vi "Generate Victim and Interferer Waveforms.vi"(6 "hardware commands sync queue":T2, 7 "measurement configuration":T1={"Victim channel"=0, "Full scale range"=10.0, "Interferer channels"=[2], "Victim channel resource name"="", "Victim frequency"=1000.0, "Victim amplitude"=-1.0, "Interferer channel resource name"="", "Interferer channel channel"=0, "Interferer start frequency"=100000.0, "Interferer stop frequency"=160000.0, "Interferer number of steps"=10, "Interferer sweep type"=0, "Interferer amplitude"=-1.0, "Digital capture resource name"="", "Digital capture sample rate"=800000.0, "Digital capture samples"=800000} {"Interferer sweep type" items=["Linear", "Logarithmic"]}, 8 "error in":errorcluster, 10 "FGen session in":refnum<k15>, 11 "DSG task in":refnum<k21>) -> (0 "error out":errorcluster)   [LabVIEW 2021, in "adc_chToChIsolationMeasurement.lvlib"]
uses:
  adc_chToChIsolationMeasurement.lvlib
  shared/controls/HW Sync Commands Queue Ref.ctl
  shared/controls/HW Sync Commands.ctl
  Measurement Configuration.ctl
  <vilib>/addons/_NISVFA/_Generation/Signal Generation/SV Signal/sv_System Timing Model.ctl
  <vilib>/DAQmx/write.llb/DAQmx Write (Analog Wfm 1Chan NSamp).vi
  <vilib>/addons/_NISVFA/_Generation/Signal Generation/SV Sinusoid/SV Sinusoid.lvclass
  C:/Program Files/National Instruments/LabVIEW 2021/vi.lib/addons/_NISVFA/_Generation/Signal Generation/SV Signal/SV Signal.lvclass
  <vilib>/addons/_NISVFA/_Generation/Signal Generation/SV Sinusoid/Configure Sine.vi
  <vilib>/addons/_NISVFA/_Generation/Signal Generation/SV Signal/Write Sample Rate.vi
  <vilib>/addons/_NISVFA/_Generation/Signal Generation/SV Signal/Write System Timing Model.vi
  <vilib>/addons/_NISVFA/_Generation/Signal Generation/SV Signal/Write Ramp Parameters.vi
  <vilib>/DAQmx/miscellaneous.llb/DAQmx Fill In Error Info.vi
  <resource>/objmgr/daqmx.rc
  <vilib>/addons/_NISVFA/_Generation/Signal Generation/SV Signal/SV Signal.lvclass
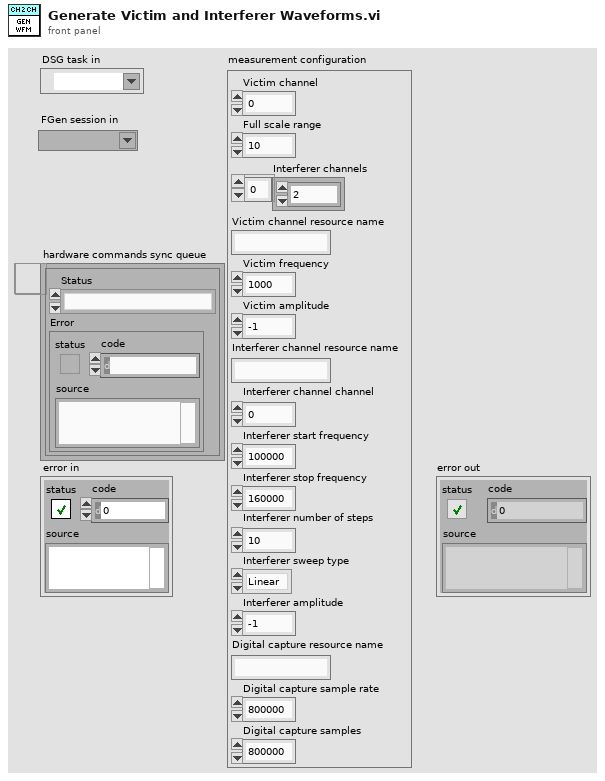
[diagram p1: front panel]
types:
  T1 = typedef "adc_chToChIsolationMeasurement.lvlib/Measurement Configuration.ctl" = cluster{"Victim channel":i32, "Full scale range":dbl, "Interferer channels":i32[], "Victim channel resource name":string, "Victim frequency":dbl, "Victim amplitude":dbl, "Interferer channel resource name":string, "Interferer channel channel":i32, "Interferer start frequency":dbl, "Interferer stop frequency":dbl, "Interferer number of steps":i32, "Interferer sweep type":u16, "Interferer amplitude":dbl, "Digital capture resource name":string, "Digital capture sample rate":dbl, "Digital capture samples":u32}
  T2 = typedef "HW Sync Commands Queue Ref.ctl" = refnum<queue>
  T3 = cluster{"profile":enum16{"Linear", "Half cosine"}, "durations [s]":cluster{"ramp-up":dbl, "transition":dbl, "ramp-down":dbl}}
  T4 = typedef "HW Sync Commands.ctl" = enum16{"NoAction", "GenerationStarted", "AcquisitionCompleted", "GenerationErrored"}
  T5 = typedef "SV Signal.lvclass/sv_System Timing Model.ctl" = i64
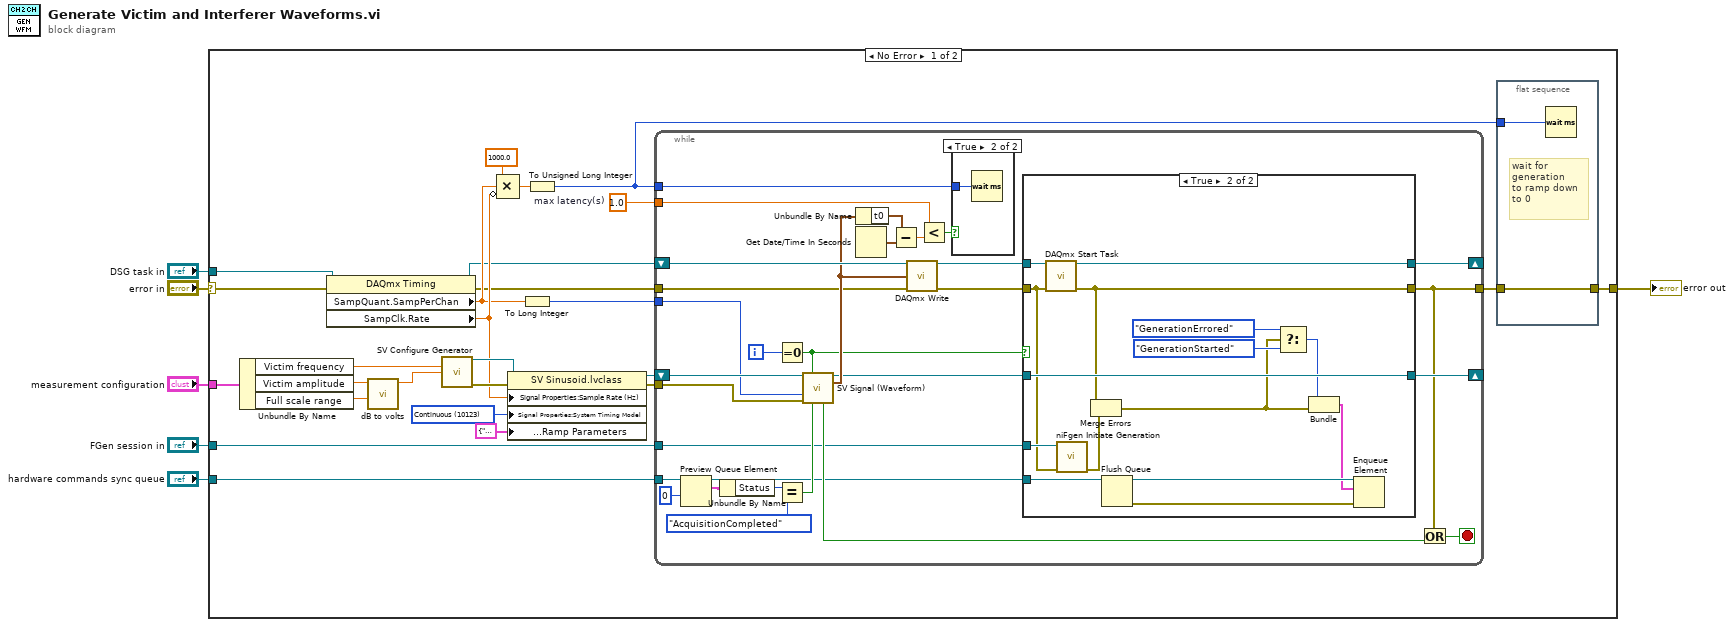
[diagram p0: block diagram]
diagram:
  n1 = case shown="No Error" "error in" {
    selector: "error in" -> [w32 w84]
    tunnel: [w31 w84] -> w5
    tunnel: "DSG task in" -> [w27 _]
    tunnel: "hardware commands sync queue" -> [w30 _]
    tunnel: "measurement configuration" -> [w29 _]
    tunnel: "FGen session in" -> [w10 _]
    frame No Error {
      w17 = 1.0  # max latency(s)
      w24 = T5 10123 items=["Finite"=10178, "-"=-1, "Continuous"=10123, "-"=-2, "Settled"=110123, "Averaged"=210123, "Discrete Sweep"=310123, "Continuous Sweep"=410123] ("System Timing Model")
      n2 = Unbundle By Name(w29) -> ("Victim frequency"=w28:dbl, "Victim amplitude"=w9:dbl, "Full scale range"=w8:dbl)
      n3 = property class="DAQmx Timing"(reference=w27, error in=w32) -> (reference out=w18:refnum<k21>, error out=w11:errorcluster, "SampQuant.SampPerChan"=w20:dbl, "SampClk.Rate"=w23:dbl)
      n4 = call "dB to volts.vi"("Full scale range"=w8, "Voltage(dB)"=w9) -> ("Voltage(volts)"=w7:dbl)  [unwired: 9 in]
      n5 = call-poly <vilib>:"SV Configure Generator.vi"("frequency (Hz)"=w28, "amplitude"=w7) -> ("signal configuration"=w25:refnum<class "SV Sinusoid.lvclass">, "error out"=w26:errorcluster)  [unwired: 12 in]
      n6 = Compound Arithmetic op=MULTIPLY(1000.0 ("value"), w20, invert w23) -> (w16:dbl)
      n7 = property class="SV Sinusoid.lvclass"(reference=w25, error in=w26, "Signal Properties:Sample Rate (Hz)"=w23, "Signal Properties:System Timing Model"=w24, "Signal Properties:Ramps:Ramp Parameters"=T3 {"profile"=enum."Linear", "durations [s]"={"ramp-up"=0.0, "transition"=0.0, "ramp-down"=0.01}} ("Ramp Parameters:All Elements")) -> (reference out=w22:refnum<class "SV Sinusoid.lvclass">, error out=w21:errorcluster)
      n8 = To Long Integer(number=w20) -> (32bit integer=w19:i32)
      n9 = To Unsigned Long Integer(number=w16) -> (unsigned 32bit integer=w13:u32)
      n10 = while {
        shift-right: [w40] -> _
        shift-left: w22 -> [w64]
        tunnel: w21 -> [w61]
        tunnel: w19 -> [w62]
        shift-right: [w43] -> _
        shift-left: w18 -> [w60]
        tunnel: [w37] -> w14
        tunnel: w17 -> [w53]
        tunnel: w13 -> [w51]
        tunnel: w30 -> [w50]
        tunnel: w11 -> [w36]
        tunnel: w10 -> [w35]
        i -> [w63]
        stop <- w58 stop-if-true
        n11 = Preview Queue Element(queue=w50, timeout in ms (-1)=0) -> (queue out=w46:T2, element=w39:cluster{"Status":T4, "Error":errorcluster})  [unwired: 1 in, 2 out]
        n12 = Unbundle By Name(w39) -> ("Status"=w38:T4)
        n13 = Equal To 0?(x=w63) -> (x = 0?=w45:bool)
        n14 = Equal?(x=w38, y=HW_Sync_Commands."AcquisitionCompleted") -> (x = y?=w47:bool)
        n15 = call-dynamic "SV Signal (Waveform).vi"("signal configuration"=w64, "reset"=w45, "samples"=w62, "error in (no error)"=w61, "stop"=w47) -> ("signal configuration"=w41:refnum<class "SV Sinusoid.lvclass">, "output waveform"=w57:waveform(dbl), "done"=w59:bool)  [unwired: 5 in, 3 out]
        n16 = Unbundle By Name(w57) -> ("t0"=w56:timestamp)
        n17 = Get Date/Time In Seconds() -> (seconds since 1Jan1904=w55:timestamp)
        n18 = Subtract(x=w56, y=w55) -> (x-y=w54:dbl)
        n19 = call-poly <vilib>:"DAQmx Write.vi"("task/channels in"=w60, "data"=w57, "error in"=w36) -> ("task out"=w44:refnum<k21>, "error out"=w42:errorcluster)  [unwired: 10 in, 1 out]
        n20 = Less?(x=w53, y=w54) -> (x < y?=w52:bool)
        n21 = case shown="True" w52 {
          tunnel: w51 -> [_ w83]
          frame False {
          }
          frame True {
            n22 = Wait (ms)(milliseconds to wait=w83) -> ()  [unwired: 1 out]
          }
        }
        n23 = case shown="True" w45 {
          tunnel: w46 -> [_ w82]
          tunnel: w44 -> [w67 w80]
          tunnel: [w67 w79] -> w43
          tunnel: w42 -> [w66 w71]
          tunnel: [w66 w69] -> w37
          tunnel: w41 -> [w65 w75]
          tunnel: [w65 w75] -> w40
          tunnel: w35 -> [_ w72]
          frame False {
          }
          frame True {
            n24 = call <vilib>:"DAQmx Start Task.vi"("task/channels in"=w80, "error in"=w71) -> ("task out"=w79:refnum<k21>, "error out"=w69:errorcluster)  [unwired: 12 in]
            n25 = call <instrlib>:"niFgen Initiate Generation.vi"("error in (no error)"=w71, "Instrument Handle"=w72) -> ("error out"=w70:errorcluster)  [unwired: 8 in, 1 out]
            n26 = Merge Errors(w69, w70) -> (w68:errorcluster)
            n27 = Flush Queue(queue=w82) -> (queue out=w81:T2, error out=w78:errorcluster)  [unwired: 1 in, 1 out]
            n28 = Select(t=HW_Sync_Commands."GenerationErrored" ("element"), s=w68, f=HW_Sync_Commands."GenerationStarted" ("element")) -> (s? t:f=w74:T4)
            n29 = Bundle("element"=w74, "error IO"=w68) -> (w73:cluster{"element":T4, "error IO":errorcluster})  [unwired: 1 in]
            n30 = Enqueue Element(queue=w81, element=w73, error in (no error)=w78) -> ()  [unwired: 1 in, 3 out]
          }
        }
        n31 = Or(x=w37, y=w59) -> (x .or. y?=w58:bool)
      }
      n32 = flat-sequence {
        tunnel: w14 -> [w34]
        tunnel: [w34] -> w31
        tunnel: w13 -> [w33]
        frame #0 {
          # "wait for\ngeneration\nto ramp down\nto 0"
          n33 = Wait (ms)(milliseconds to wait=w33) -> ()  [unwired: 1 out]
        }
      }
    }
    frame Error {
    }
  }
  "error out" <- w5
